vi "Labview5_1.vi"() -> ()   [LabVIEW 2015]
panel:
  out "LED3":bool
  out "LED2":bool
  out "LED1":bool
  in  "Sequence LEDs":bool
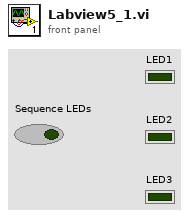
[diagram p1: front panel]
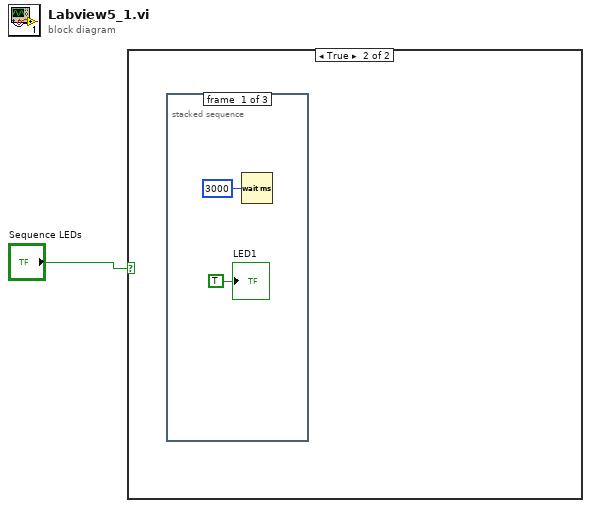
[diagram p0: block diagram]
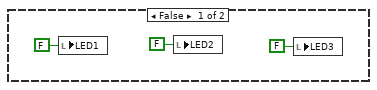
[diagram p2: hidden frame]
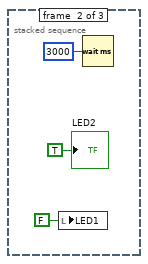
[diagram p3: hidden frame]
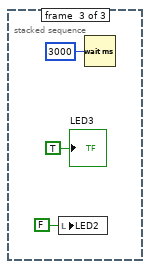
[diagram p4: hidden frame]
diagram:
  n1 = case shown="True" "Sequence LEDs" {
    frame False {
      n2 = local write "LED1"(FALSE ("LED1")) -> ()
      n3 = local write "LED2"(FALSE ("LED2")) -> ()
      n4 = local write "LED3"(FALSE ("LED3")) -> ()
    }
    frame True {
      n5 = stacked-sequence {
        frame #0 {
          n6 = Wait (ms)(milliseconds to wait=u32 3000) -> ()  [unwired: 1 out]
          "LED1" <- TRUE ("LED1")
        }
        frame #1 {
          n7 = local write "LED1"(FALSE ("LED1")) -> ()
          n8 = Wait (ms)(milliseconds to wait=u32 3000) -> ()  [unwired: 1 out]
          "LED2" <- TRUE ("LED2")
        }
        frame #2 {
          n9 = local write "LED2"(FALSE ("LED2")) -> ()
          n10 = Wait (ms)(milliseconds to wait=u32 3000) -> ()  [unwired: 1 out]
          "LED3" <- TRUE ("LED3")
        }
      }
    }
  }
